vi "Test Regex Finder.vi"(11 "Test Case In":refnum<class "Date Regex Finder Tests.lvclass">) -> (0 "error out":errorcluster, 3 "Test Case Out":refnum<class "Date Regex Finder Tests.lvclass">)   [LabVIEW 2020, in "Date Regex Finder Tests.lvclass"]
uses:
  Date Regex Finder Tests.lvclass
  C:/Program Files/National Instruments/LabVIEW 2026/vi.lib/Astemes/LUnit/Test Case.lvclass
  Date Regex Finder Tests.lvclass/Date Regex Finder Tests.ctl
  <vilib>/Astemes/LUnit/Test Case.lvclass/Test Case.ctl
  4993e8ee-a06a-463a-9684-69129f64d5ce.vi
  <vilib>/Astemes/LUnit/Core/LUnit Test Case/Private/Append Pass Result.vi
  <vilib>/Astemes/LUnit/Core/LUnit Test Case/Private/Append Fail Result.vi
  4993e8ee-a06a-463a-9684-69129f64d5ce.vi/9c5d11cd-9439-4240-a1ee-d9baace9c924.vi
  <vilib>/Astemes/LUnit/Core/LUnit Test Case/Private/Run In UI.vi
  <vilib>/Utility/error.llb/Clear Errors.vi
  Source/Approval Tests/Date Scrubber/Date Scrubber.lvclass
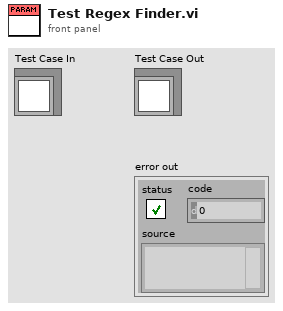
[diagram p1: front panel]
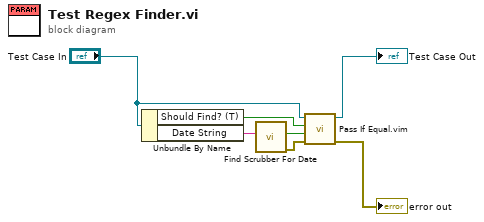
[diagram p0: block diagram]
diagram:
  n1 = Unbundle By Name("Test Case In") -> ("Should Find? (T)"=w3:bool, "Date String"=w2:string)
  n2 = call "Find Scrubber For Date.vi"("Sample Date"=w2) -> ("error out"=w6:errorcluster, "Found?"=w1:bool)  [unwired: 8 in, 1 out]
  n3 = call "Pass If Equal.vim"("error in (no error)"=w6, "Actual"=w1, "Expected"=w3, "LUnit Test Case In"="Test Case In") -> ("error out"=→"error out":errorcluster, "LUnit Test Case Out"=→"Test Case Out":refnum<class "Date Regex Finder Tests.lvclass">)  [unwired: 6 in]
